vi "Write Number of Tatics.vi"(8 "error in (no error)":errorcluster, 10 "Number of Tatics":dbl, 11 "SimplePassReceiverRole in":refnum<class "SimplePassReceiverRole.lvclass">) -> (0 "error out":errorcluster, 3 "SimplePassReceiverRole out":refnum<class "SimplePassReceiverRole.lvclass">)   [LabVIEW 2021, in "SimplePassReceiverRole.lvclass"]
uses:
  SimplePassReceiverRole.lvclass
  SimplePassReceiverRole.lvclass/SimplePassReceiverRole.ctl
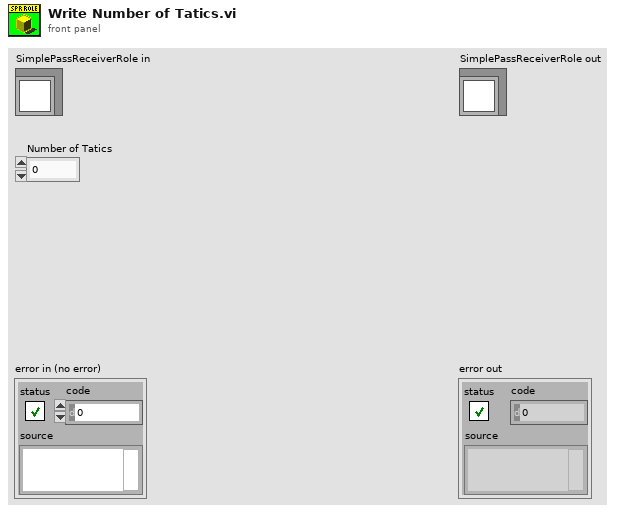
[diagram p1: front panel]
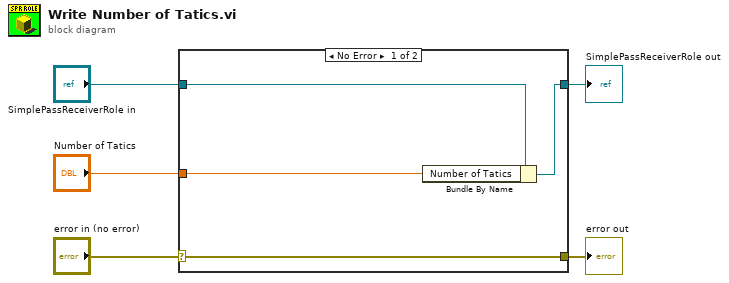
[diagram p0: block diagram]
diagram:
  n1 = case shown="No Error" "error in (no error)" {
    selector: "error in (no error)" -> [w9 w10]
    tunnel: [w9 w10] -> w4
    tunnel: [w7 w11] -> w2
    tunnel: "SimplePassReceiverRole in" -> [w8 w11]
    tunnel: "Number of Tatics" -> [w6 _]
    frame No Error {
      n2 = Bundle By Name(cluster=w8, "Number of Tatics"=w6) -> (w7:refnum<class "SimplePassReceiverRole.lvclass">)
    }
    frame Error {
    }
  }
  "error out" <- w4
  "SimplePassReceiverRole out" <- w2
